vi "Get Legend Color.vi"(9 "Pair Array Length":i32, 11 "Color Pair Array In":cluster{"Color":u32, "String":string}[](array[cluster])) -> (3 "Color Pair Array Out":cluster{"Color":u32, "String":string}[](array[cluster]))   [LabVIEW 2020, in "3D Plot.lvclass"]
uses:
  <vilib>/Math Plots/3D Math Plots/3D Plot/3D Plot/3D Plot.lvclass
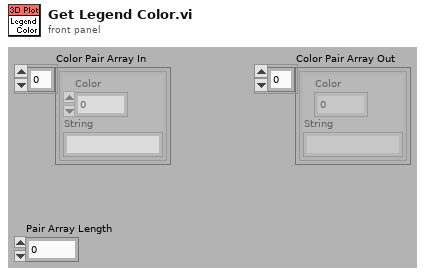
[diagram p1: front panel]
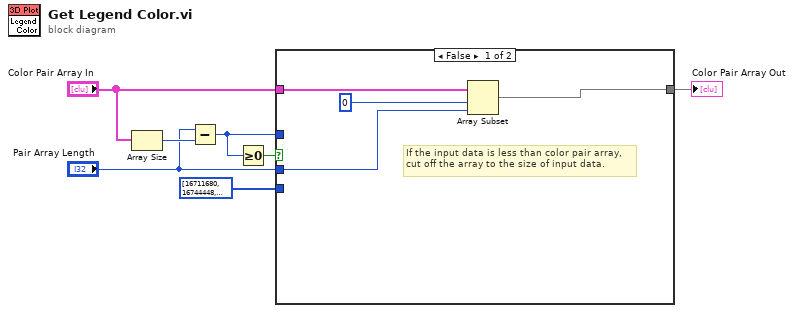
[diagram p0: block diagram]
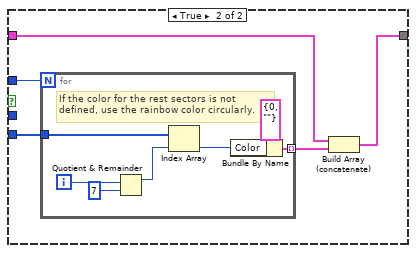
[diagram p2: hidden frame]
diagram:
  n1 = Array Size(array="Color Pair Array In") -> (size(s)=w7:i32)
  n2 = Subtract(x="Pair Array Length", y=w7) -> (x-y=w5:i32)
  n3 = Greater Or Equal To 0?(x=w5) -> (x >= 0?=w4:bool)
  n4 = case shown="False" w4 {
    tunnel: u32[] [16711680, 16744448, 16776960, 65280, 65535, 255, 8388736] ("appended array") -> [_ w16]
    tunnel: w5 -> [_ w15]
    tunnel: "Pair Array Length" -> [w9 _]
    tunnel: "Color Pair Array In" -> [w11 w14]
    tunnel: [w10 w12] -> w1
    frame False {
      # "If the input data is less than color pair array,\ncut off the array to the size of input data."
      n5 = Array Subset(array=w11, index=0, length=w9) -> (w10:cluster{"Color":u32, "String":string}[])
    }
    frame True {
      n6 = for {
        N: w15 -> [_]
        tunnel: w16 -> [w23]
        tunnel: [w22] -> w13 mode=indexing
        i -> [w17]
        # "If the color for the rest sectors is not\ndefined, use the rainbow color circularly."
        n7 = Quotient & Remainder(x=w17, y=7) -> (x-y*floor(x/y)=w21:i32)  [unwired: 1 out]
        n8 = Index Array(array=w23, index=w21) -> (element=w18:u32)
        n9 = Bundle By Name(cluster=cluster{"Color":u32, "String":string} {"Color"=0, "String"=""} ("element"), "Color"=w18) -> (w22:cluster{"Color":u32, "String":string})
      }
      n10 = Build Array (concatenate)(w14, w13) -> (w12:cluster{"Color":u32, "String":string}[])
    }
  }
  "Color Pair Array Out" <- w1
